vi "S4ICS Batch Command.vi"() -> ()   [LabVIEW 2018]
panel:
  out "cmd #":i32
  out "current time":timestamp format="%<%H:%M:%S%3u\n%Y/%m/%d>T"
  out "batch cmd":string
  in  "batch file":string="WPROT" caption="Batch File Name"
  in  "allin":T1={"s4icsIP"="localhost", "s4icsPort"=54165, "mech name"="", "cmd"=[], "log"=refnum} {"s4icsPort" min=1025 step=1}
  in  "stop":bool
  # "S4ICS Batch Command"
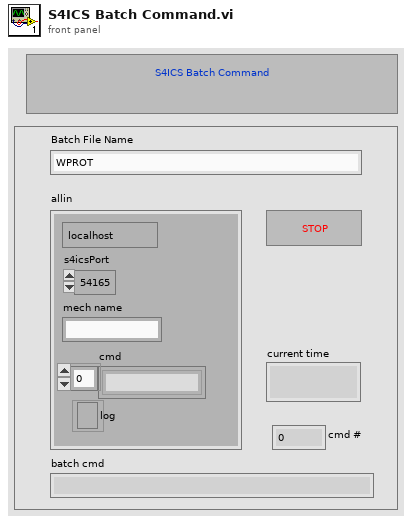
[diagram p1: front panel]
types:
  T1 = cluster{"s4icsIP":string, "s4icsPort":u16, "mech name":string, "cmd":string[], "log":refnum<file>}
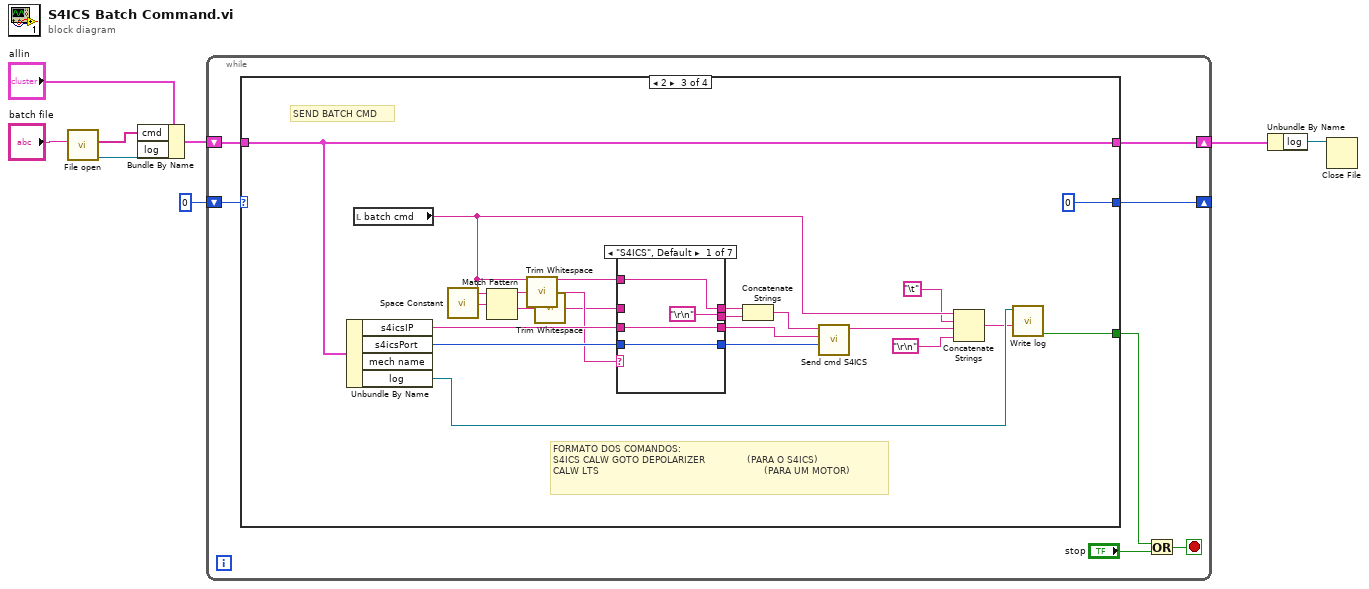
[diagram p0: block diagram]
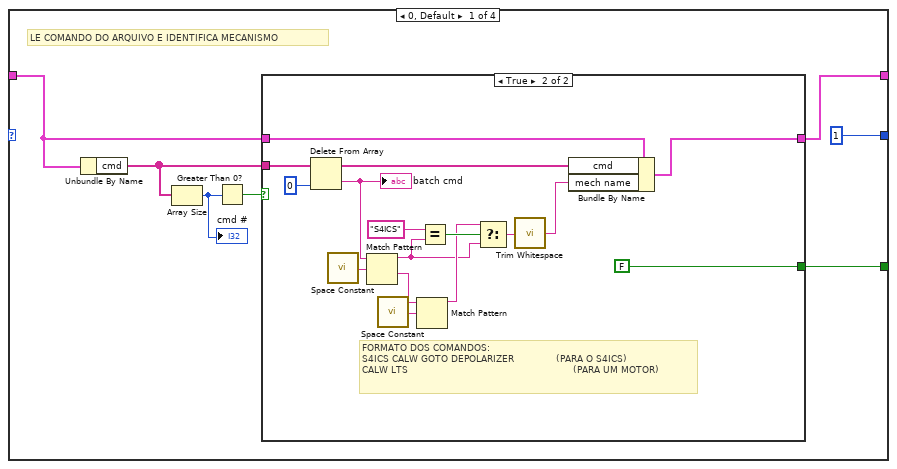
[diagram p2: hidden frame]
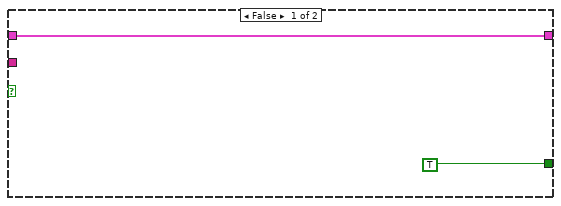
[diagram p3: hidden frame]
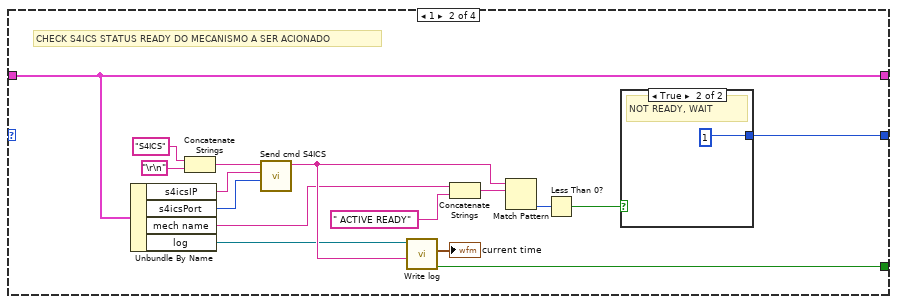
[diagram p4: hidden frame]
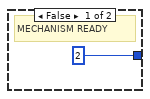
[diagram p5: hidden frame]
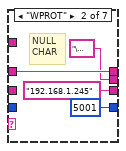
[diagram p6: hidden frame]
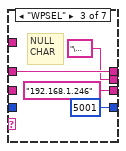
[diagram p7: hidden frame]
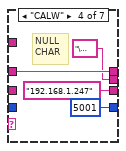
[diagram p8: hidden frame]
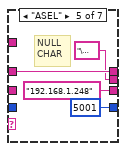
[diagram p9: hidden frame]
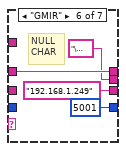
[diagram p10: hidden frame]
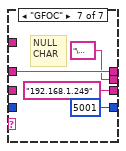
[diagram p11: hidden frame]
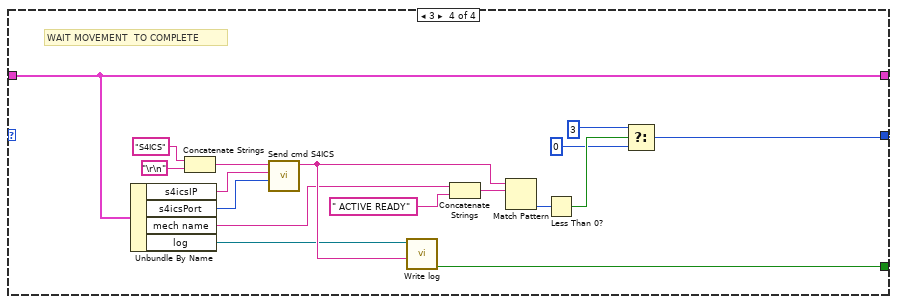
[diagram p12: hidden frame]
diagram:
  n1 = call "File open.vi"("file name"="batch file") -> ("log"=w5:refnum<file>, "cmd"=w4:string[])  [unwired: 9 in]
  n2 = Bundle By Name(cluster="allin", "cmd"=w4, "log"=w5) -> (w6:T1)
  n3 = while {
    shift-right: [w14] -> _
    shift-left: u8 0 -> [w15]
    shift-right: [w12] -> w2
    shift-left: w6 -> [w13]
    stop <- w10 stop-if-true
    n4 = case shown="2" w15 {
      tunnel: [u8 1 ("x+1") w41 u8 0 ("x+1") w123] -> w14
      tunnel: w13 -> [w20 w49 w77 w124]
      tunnel: [w17 w49 w77 w124] -> w12
      tunnel: [w19 w47 w68 w122] -> w9
      frame 0, Default {
        # "LE COMANDO DO ARQUIVO E IDENTIFICA MECANISMO"
        n5 = Unbundle By Name(w20) -> ("cmd"=w16:string[])
        n6 = Array Size(array=w16) -> (size(s)=w22:i32)
        "cmd #" <- w22
        n7 = Greater Than 0?(x=w22) -> (x > 0?=w21:bool)
        n8 = case shown="True" w21 {
          tunnel: w16 -> [_ w40]
          tunnel: w20 -> [w24 w39]
          tunnel: [w24 w38] -> w17
          tunnel: [TRUE FALSE] -> w19
          frame False {
          }
          frame True {
            # "FORMATO DOS COMANDOS:\nS4ICS CALW GOTO DEPOLARIZER              (PARA O S4ICS)\nCALW LTS                                                       (PARA UM MOTOR)"
            n9 = Delete From Array(array=w40, index=0) -> (deleted portion=w34:string, array with subset deleted=w37:string[])  [unwired: 1 in]
            "batch cmd" <- w34
            n10 = call <vilib>:"Space Constant.vi"() -> ("String"=w35:string)
            n11 = Match Pattern(string=w34, regular expression=w35) -> (before substring=w27:string, after substring=w31:string)  [unwired: 1 in, 2 out]
            n12 = call <vilib>:"Space Constant.vi"() -> ("String"=w32:string)
            n13 = Match Pattern(string=w31, regular expression=w32) -> (before substring=w28:string)  [unwired: 1 in, 3 out]
            n14 = Equal?(x="S4ICS", y=w27) -> (x = y?=w29:bool)
            n15 = Select(t=w28, s=w29, f=w27) -> (s? t:f=w26:string)
            n16 = call <vilib>:"Trim Whitespace.vi"("string"=w26) -> ("trimmed string"=w25:string)  [unwired: 1 in]
            n17 = Bundle By Name(cluster=w39, "cmd"=w37, "mech name"=w25) -> (w38:T1)
          }
        }
      }
      frame 1 {
        # "CHECK S4ICS STATUS READY DO MECANISMO A SER ACIONADO"
        n18 = Unbundle By Name(w49) -> ("s4icsIP"=w54:string, "s4icsPort"=w53:u16, "mech name"=w44:string, "log"=w46:refnum<file>)
        n19 = Concatenate Strings("S4ICS", "\r\n") -> (w52:string)
        n20 = call "Send cmd S4ICS.vi"("port"=w53, "address"=w54, "data in"=w52) -> ("data out"=w48:string)  [unwired: 7 in, 1 out]
        n21 = call "Write log.vi"("text"=w48, "log file"=w46) -> ("status"=w47:bool, "current time"=→"current time":timestamp)  [unwired: 8 in]
        n22 = Concatenate Strings(w44, " ACTIVE READY") -> (w45:string)
        n23 = Match Pattern(string=w48, regular expression=w45) -> (offset past match=w51:i32)  [unwired: 1 in, 3 out]
        n24 = Less Than 0?(x=w51) -> (x < 0?=w42:bool)
        n25 = case shown="True" w42 {
          tunnel: [u8 2 ("f") u8 1 ("f")] -> w41
          frame False {
            # "MECHANISM READY"
          }
          frame True {
            # "NOT READY, WAIT"
          }
        }
      }
      frame 2 {
        # "FORMATO DOS COMANDOS:\nS4ICS CALW GOTO DEPOLARIZER              (PARA O S4ICS)\nCALW LTS                                                       (PARA UM MOTOR)"
        # "SEND BATCH CMD"
        n26 = Unbundle By Name(w77) -> ("s4icsIP"=w79:string, "s4icsPort"=w78:u16, "log"=w67:refnum<file>)  [unwired: 1 out]
        n27 = local read "batch cmd"() -> (w66:string)
        n28 = call <vilib>:"Space Constant.vi"() -> ("String"=w72:string)
        n29 = Match Pattern(string=w66, regular expression=w72) -> (before substring=w62:string, after substring=w71:string)  [unwired: 1 in, 2 out]
        n30 = call <vilib>:"Trim Whitespace.vi"("string"=w62) -> ("trimmed string"=w61:string)  [unwired: 1 in]
        n31 = call <vilib>:"Trim Whitespace.vi"("string"=w71) -> ("trimmed string"=w60:string)  [unwired: 1 in]
        n32 = case shown="\"S4ICS\", Default" w61 {
          tunnel: w79 -> [w83 _ _ _ _ _ _]
          tunnel: w78 -> [w82 _ _ _ _ _ _]
          tunnel: [w83 "192.168.1.245" ("s4icsIP") "192.168.1.246" ("s4icsIP") "192.168.1.247" ("s4icsIP") "192.168.1.248" ("s4icsIP") "192.168.1.249" ("s4icsIP") "192.168.1.249" ("s4icsIP")] -> w75
          tunnel: [w82 u16 5001 ("s4icsPort") u16 5001 ("s4icsPort") u16 5001 ("s4icsPort") u16 5001 ("s4icsPort") u16 5001 ("s4icsPort") u16 5001 ("s4icsPort")] -> w74
          tunnel: w60 -> [_ w85 w89 w93 w97 w101 w105]
          tunnel: w66 -> [w81 _ _ _ _ _ _]
          tunnel: [w81 w85 w89 w93 w97 w101 w105] -> w70
          tunnel: ["\r\n" "\u0000" ("search string") "\u0000" ("search string") "\u0000" ("search string") "\u0000" ("search string") "\u0000" ("search string") "\u0000" ("search string")] -> w69
          frame "S4ICS", Default {
          }
          frame "WPROT" {
            # "NULL\nCHAR"
          }
          frame "WPSEL" {
            # "NULL\nCHAR"
          }
          frame "CALW" {
            # "NULL\nCHAR"
          }
          frame "ASEL" {
            # "NULL\nCHAR"
          }
          frame "GMIR" {
            # "NULL\nCHAR"
          }
          frame "GFOC" {
            # "NULL\nCHAR"
          }
        }
        n33 = Concatenate Strings(w70, w69) -> (w73:string)
        n34 = call "Send cmd S4ICS.vi"("port"=w74, "address"=w75, "data in"=w73) -> ("data out"=w65:string)  [unwired: 7 in, 1 out]
        n35 = Concatenate Strings(w66, "\t", w65, "\r\n") -> (w64:string)
        n36 = call "Write log.vi"("text"=w64, "log file"=w67) -> ("status"=w68:bool)  [unwired: 8 in, 1 out]
      }
      frame 3 {
        # "WAIT MOVEMENT  TO COMPLETE"
        n37 = Unbundle By Name(w124) -> ("s4icsIP"=w119:string, "s4icsPort"=w118:u16, "mech name"=w109:string, "log"=w111:refnum<file>)
        n38 = Concatenate Strings("S4ICS", "\r\n") -> (w117:string)
        n39 = call "Send cmd S4ICS.vi"("port"=w118, "address"=w119, "data in"=w117) -> ("data out"=w112:string)  [unwired: 7 in, 1 out]
        n40 = call "Write log.vi"("text"=w112, "log file"=w111) -> ("status"=w122:bool)  [unwired: 8 in, 1 out]
        n41 = Concatenate Strings(w109, " ACTIVE READY") -> (w110:string)
        n42 = Match Pattern(string=w112, regular expression=w110) -> (offset past match=w116:i32)  [unwired: 1 in, 3 out]
        n43 = Less Than 0?(x=w116) -> (x < 0?=w114:bool)
        n44 = Select(t=u8 3 ("f"), s=w114, f=u8 0) -> (s? t:f=w123:u8)
      }
    }
    n45 = Or(x=w9, y="stop") -> (x .or. y?=w10:bool)
  }
  n46 = Unbundle By Name(w2) -> ("log"=w1:refnum<file>)
  n47 = Close File(refnum=w1) -> ()  [unwired: 1 in, 2 out]
